vi "Pre Launch Init.vi"(11 "UDP_Service in":refnum<class "UDP_Service.lvclass">) -> (0 "error out":errorcluster, 3 "UDP_Service out":refnum<class "UDP_Service.lvclass">)   [LabVIEW 2016, in "CoreAssertAPI.lvlib" / "UDP_Service.lvclass"]
doc: "(<B>Filename</B>: Actor Framework.lvlib:Actor.lvclass:Pre Launch Init.vi)\n\nDefines behavior that occurs after the Launch Nested Actor method is invoked but before the actor's Actor Core method begins running.\n\nBy default, this method does nothing. A descendant class may override it to define behavior."
uses:
  UDP_Service.lvclass
  UDP_Service.lvclass/UDP_Service.ctl
  <vilib>/ActorFramework/Actor/Actor.lvclass
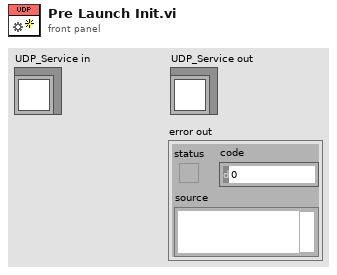
[diagram p1: front panel]
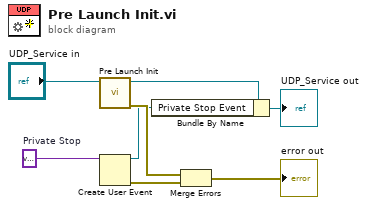
[diagram p0: block diagram]
diagram:
  w5 = variant  # Private Stop
  n1 = call-parent "Pre Launch Init.vi"("Actor in"="UDP_Service in") -> ("error out"=w6:errorcluster, "Actor out"=w8:refnum<class "UDP_Service.lvclass">)  [unwired: 9 in]
  n2 = Create User Event(user event datatype=w5) -> (user event=w3:refnum<user-event>, error out=w1:errorcluster)  [unwired: 1 in]
  n3 = Bundle By Name(cluster=w8, "Private Stop Event"=w3) -> (→"UDP_Service out":refnum<class "UDP_Service.lvclass">)
  n4 = Merge Errors(w6, w1) -> (→"error out":errorcluster)
